vi "Waveform N channels LP pt by pt prefilter.vi"(6 "order":i32=2, 8 "fl":dbl, 10 "fs":dbl, 11 "Array in":waveform(dbl)[](array[waveform])) -> (3 "Array out":waveform(dbl)[](array[waveform]))   [LabVIEW 2013]
uses:
  <vilib>/Analysis/3filter.llb/Filter Passband Type.ctl
  <vilib>/ptbypt/NI_PtbyPt.lvlib
  <vilib>/Analysis/NI_AALBase.lvlib
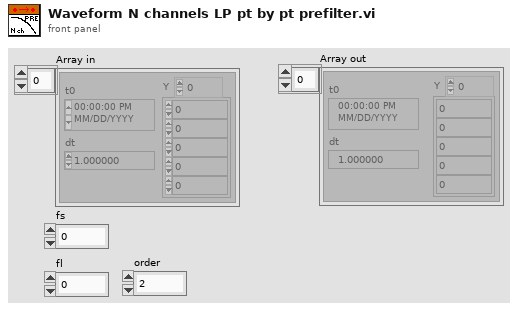
[diagram p1: front panel]
types:
  T1 = typedef "NI_AALBase.lvlib/Filter Passband Type.ctl" = enum32{"Lowpass", "Highpass", "Bandpass", "Bandstop"}
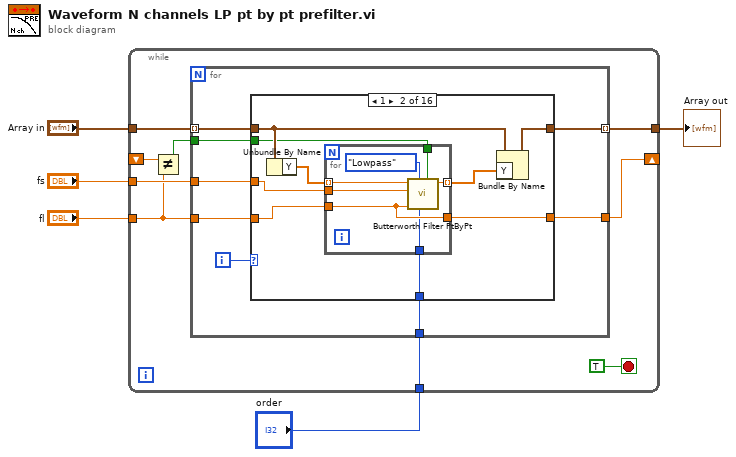
[diagram p0: block diagram]
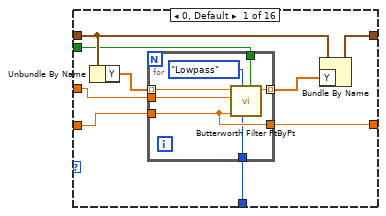
[diagram p2: hidden frame]
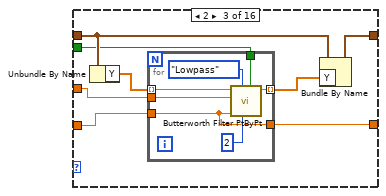
[diagram p3: hidden frame]
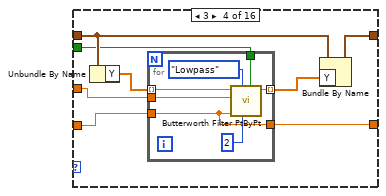
[diagram p4: hidden frame]
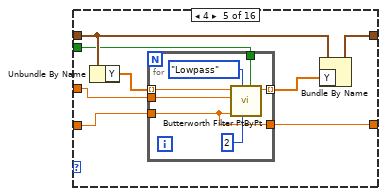
[diagram p5: hidden frame]
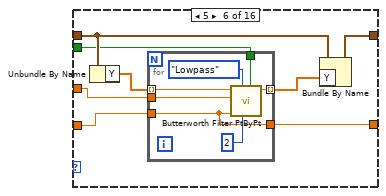
[diagram p6: hidden frame]
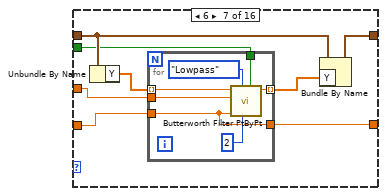
[diagram p7: hidden frame]
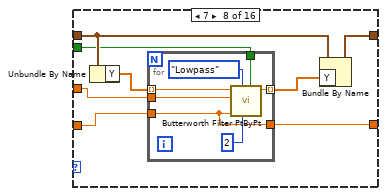
[diagram p8: hidden frame]
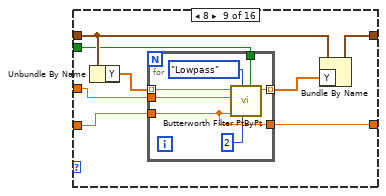
[diagram p9: hidden frame]
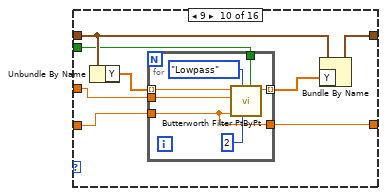
[diagram p10: hidden frame]
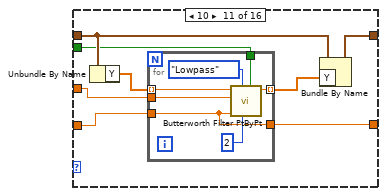
[diagram p11: hidden frame]
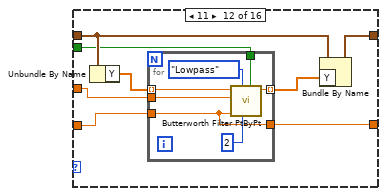
[diagram p12: hidden frame]
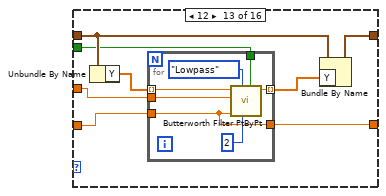
[diagram p13: hidden frame]
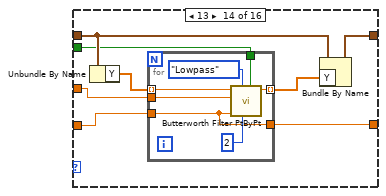
[diagram p14: hidden frame]
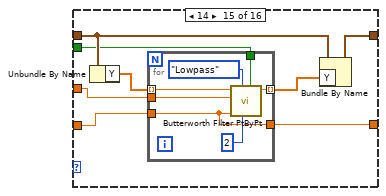
[diagram p15: hidden frame]
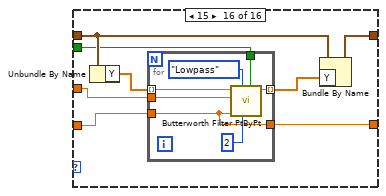
[diagram p16: hidden frame]
diagram:
  n1 = while {
    tunnel: "Array in" -> [w14]
    tunnel: [w13] -> w4
    tunnel: "fs" -> [w10]
    tunnel: "fl" -> [w7]
    shift-right: [w11] -> _
    shift-left: _ -> [w9]
    tunnel: "order" -> [w8]
    stop <- TRUE stop-if-true
    n2 = Not Equal?(x=w9, y=w7) -> (x != y?=w6:bool)
    n3 = for {
      tunnel: w14 -> [w20] mode=indexing
      tunnel: w10 -> [w22]
      tunnel: [w21] -> w13 mode=indexing
      tunnel: w7 -> [w19]
      tunnel: [w17] -> w11
      tunnel: w6 -> [w16]
      tunnel: w8 -> [w15]
      i -> [w18]
      n4 = case shown="1" w18 {
        tunnel: w22 -> [w27 w43 w58 w73 w88 w103 w118 w133 w148 w163 w178 w193 w208 w223 w238 w253]
        tunnel: [w31 w47 w62 w77 w92 w107 w122 w137 w152 w167 w182 w197 w212 w227 w242 w257] -> w21
        tunnel: w20 -> [w29 w45 w60 w75 w90 w105 w120 w135 w150 w165 w180 w195 w210 w225 w240 w255]
        tunnel: [w30 w46 w61 w76 w91 w106 w121 w136 w151 w166 w181 w196 w211 w226 w241 w256] -> w17
        tunnel: w19 -> [w26 w42 w57 w72 w87 w102 w117 w132 w147 w162 w177 w192 w207 w222 w237 w252]
        tunnel: w16 -> [w24 w40 w55 w70 w85 w100 w115 w130 w145 w160 w175 w190 w205 w220 w235 w250]
        tunnel: w15 -> [w23 w39 _ _ _ _ _ _ _ _ _ _ _ _ _ _]
        frame 0, Default {
          n5 = Unbundle By Name(w29) -> ("Y"=w25:dbl[])
          n6 = for {
            tunnel: w25 -> [w38] mode=indexing
            tunnel: w26 -> [w35]
            tunnel: w27 -> [w37]
            tunnel: [w36] -> w28 mode=indexing
            tunnel: [w35] -> w30
            tunnel: w24 -> [w33]
            tunnel: w23 -> [w32]
            n7 = call <vilib>:"Butterworth Filter PtByPt.vi"("initialize"=w33, "order"=w32, "filter type"=Filter_Passband_Type."Lowpass", "low cutoff freq: fl"=w35, "sampling freq: fs"=w37, "x"=w38) -> ("Filtered x"=w36:dbl)  [unwired: 3 in, 1 out]
          }
          n8 = Bundle By Name(cluster=w29, "Y"=w28) -> (w31:waveform(dbl))
        }
        frame 1 {
          n9 = Unbundle By Name(w45) -> ("Y"=w41:dbl[])
          n10 = for {
            tunnel: w41 -> [w54] mode=indexing
            tunnel: w42 -> [w51]
            tunnel: w43 -> [w53]
            tunnel: [w52] -> w44 mode=indexing
            tunnel: [w51] -> w46
            tunnel: w40 -> [w49]
            tunnel: w39 -> [w48]
            n11 = call <vilib>:"Butterworth Filter PtByPt.vi"("initialize"=w49, "order"=w48, "filter type"=Filter_Passband_Type."Lowpass", "low cutoff freq: fl"=w51, "sampling freq: fs"=w53, "x"=w54) -> ("Filtered x"=w52:dbl)  [unwired: 3 in, 1 out]
          }
          n12 = Bundle By Name(cluster=w45, "Y"=w44) -> (w47:waveform(dbl))
        }
        frame 2 {
          n13 = Unbundle By Name(w60) -> ("Y"=w56:dbl[])
          n14 = for {
            tunnel: w56 -> [w69] mode=indexing
            tunnel: w57 -> [w65]
            tunnel: w58 -> [w67]
            tunnel: [w66] -> w59 mode=indexing
            tunnel: [w65] -> w61
            tunnel: w55 -> [w63]
            n15 = call <vilib>:"Butterworth Filter PtByPt.vi"("initialize"=w63, "order"=2, "filter type"=Filter_Passband_Type."Lowpass", "low cutoff freq: fl"=w65, "sampling freq: fs"=w67, "x"=w69) -> ("Filtered x"=w66:dbl)  [unwired: 3 in, 1 out]
          }
          n16 = Bundle By Name(cluster=w60, "Y"=w59) -> (w62:waveform(dbl))
        }
        frame 3 {
          n17 = Unbundle By Name(w75) -> ("Y"=w71:dbl[])
          n18 = for {
            tunnel: w71 -> [w84] mode=indexing
            tunnel: w72 -> [w80]
            tunnel: w73 -> [w82]
            tunnel: [w81] -> w74 mode=indexing
            tunnel: [w80] -> w76
            tunnel: w70 -> [w78]
            n19 = call <vilib>:"Butterworth Filter PtByPt.vi"("initialize"=w78, "order"=2, "filter type"=Filter_Passband_Type."Lowpass", "low cutoff freq: fl"=w80, "sampling freq: fs"=w82, "x"=w84) -> ("Filtered x"=w81:dbl)  [unwired: 3 in, 1 out]
          }
          n20 = Bundle By Name(cluster=w75, "Y"=w74) -> (w77:waveform(dbl))
        }
        frame 4 {
          n21 = Unbundle By Name(w90) -> ("Y"=w86:dbl[])
          n22 = for {
            tunnel: w86 -> [w99] mode=indexing
            tunnel: w87 -> [w95]
            tunnel: w88 -> [w97]
            tunnel: [w96] -> w89 mode=indexing
            tunnel: [w95] -> w91
            tunnel: w85 -> [w93]
            n23 = call <vilib>:"Butterworth Filter PtByPt.vi"("initialize"=w93, "order"=2, "filter type"=Filter_Passband_Type."Lowpass", "low cutoff freq: fl"=w95, "sampling freq: fs"=w97, "x"=w99) -> ("Filtered x"=w96:dbl)  [unwired: 3 in, 1 out]
          }
          n24 = Bundle By Name(cluster=w90, "Y"=w89) -> (w92:waveform(dbl))
        }
        frame 5 {
          n25 = Unbundle By Name(w105) -> ("Y"=w101:dbl[])
          n26 = for {
            tunnel: w101 -> [w114] mode=indexing
            tunnel: w102 -> [w110]
            tunnel: w103 -> [w112]
            tunnel: [w111] -> w104 mode=indexing
            tunnel: [w110] -> w106
            tunnel: w100 -> [w108]
            n27 = call <vilib>:"Butterworth Filter PtByPt.vi"("initialize"=w108, "order"=2, "filter type"=Filter_Passband_Type."Lowpass", "low cutoff freq: fl"=w110, "sampling freq: fs"=w112, "x"=w114) -> ("Filtered x"=w111:dbl)  [unwired: 3 in, 1 out]
          }
          n28 = Bundle By Name(cluster=w105, "Y"=w104) -> (w107:waveform(dbl))
        }
        frame 6 {
          n29 = Unbundle By Name(w120) -> ("Y"=w116:dbl[])
          n30 = for {
            tunnel: w116 -> [w129] mode=indexing
            tunnel: w117 -> [w125]
            tunnel: w118 -> [w127]
            tunnel: [w126] -> w119 mode=indexing
            tunnel: [w125] -> w121
            tunnel: w115 -> [w123]
            n31 = call <vilib>:"Butterworth Filter PtByPt.vi"("initialize"=w123, "order"=2, "filter type"=Filter_Passband_Type."Lowpass", "low cutoff freq: fl"=w125, "sampling freq: fs"=w127, "x"=w129) -> ("Filtered x"=w126:dbl)  [unwired: 3 in, 1 out]
          }
          n32 = Bundle By Name(cluster=w120, "Y"=w119) -> (w122:waveform(dbl))
        }
        frame 7 {
          n33 = Unbundle By Name(w135) -> ("Y"=w131:dbl[])
          n34 = for {
            tunnel: w131 -> [w144] mode=indexing
            tunnel: w132 -> [w140]
            tunnel: w133 -> [w142]
            tunnel: [w141] -> w134 mode=indexing
            tunnel: [w140] -> w136
            tunnel: w130 -> [w138]
            n35 = call <vilib>:"Butterworth Filter PtByPt.vi"("initialize"=w138, "order"=2, "filter type"=Filter_Passband_Type."Lowpass", "low cutoff freq: fl"=w140, "sampling freq: fs"=w142, "x"=w144) -> ("Filtered x"=w141:dbl)  [unwired: 3 in, 1 out]
          }
          n36 = Bundle By Name(cluster=w135, "Y"=w134) -> (w137:waveform(dbl))
        }
        frame 8 {
          n37 = Unbundle By Name(w150) -> ("Y"=w146:dbl[])
          n38 = for {
            tunnel: w146 -> [w159] mode=indexing
            tunnel: w147 -> [w155]
            tunnel: w148 -> [w157]
            tunnel: [w156] -> w149 mode=indexing
            tunnel: [w155] -> w151
            tunnel: w145 -> [w153]
            n39 = call <vilib>:"Butterworth Filter PtByPt.vi"("initialize"=w153, "order"=2, "filter type"=Filter_Passband_Type."Lowpass", "low cutoff freq: fl"=w155, "sampling freq: fs"=w157, "x"=w159) -> ("Filtered x"=w156:dbl)  [unwired: 3 in, 1 out]
          }
          n40 = Bundle By Name(cluster=w150, "Y"=w149) -> (w152:waveform(dbl))
        }
        frame 9 {
          n41 = Unbundle By Name(w165) -> ("Y"=w161:dbl[])
          n42 = for {
            tunnel: w161 -> [w174] mode=indexing
            tunnel: w162 -> [w170]
            tunnel: w163 -> [w172]
            tunnel: [w171] -> w164 mode=indexing
            tunnel: [w170] -> w166
            tunnel: w160 -> [w168]
            n43 = call <vilib>:"Butterworth Filter PtByPt.vi"("initialize"=w168, "order"=2, "filter type"=Filter_Passband_Type."Lowpass", "low cutoff freq: fl"=w170, "sampling freq: fs"=w172, "x"=w174) -> ("Filtered x"=w171:dbl)  [unwired: 3 in, 1 out]
          }
          n44 = Bundle By Name(cluster=w165, "Y"=w164) -> (w167:waveform(dbl))
        }
        frame 10 {
          n45 = Unbundle By Name(w180) -> ("Y"=w176:dbl[])
          n46 = for {
            tunnel: w176 -> [w189] mode=indexing
            tunnel: w177 -> [w185]
            tunnel: w178 -> [w187]
            tunnel: [w186] -> w179 mode=indexing
            tunnel: [w185] -> w181
            tunnel: w175 -> [w183]
            n47 = call <vilib>:"Butterworth Filter PtByPt.vi"("initialize"=w183, "order"=2, "filter type"=Filter_Passband_Type."Lowpass", "low cutoff freq: fl"=w185, "sampling freq: fs"=w187, "x"=w189) -> ("Filtered x"=w186:dbl)  [unwired: 3 in, 1 out]
          }
          n48 = Bundle By Name(cluster=w180, "Y"=w179) -> (w182:waveform(dbl))
        }
        frame 11 {
          n49 = Unbundle By Name(w195) -> ("Y"=w191:dbl[])
          n50 = for {
            tunnel: w191 -> [w204] mode=indexing
            tunnel: w192 -> [w200]
            tunnel: w193 -> [w202]
            tunnel: [w201] -> w194 mode=indexing
            tunnel: [w200] -> w196
            tunnel: w190 -> [w198]
            n51 = call <vilib>:"Butterworth Filter PtByPt.vi"("initialize"=w198, "order"=2, "filter type"=Filter_Passband_Type."Lowpass", "low cutoff freq: fl"=w200, "sampling freq: fs"=w202, "x"=w204) -> ("Filtered x"=w201:dbl)  [unwired: 3 in, 1 out]
          }
          n52 = Bundle By Name(cluster=w195, "Y"=w194) -> (w197:waveform(dbl))
        }
        frame 12 {
          n53 = Unbundle By Name(w210) -> ("Y"=w206:dbl[])
          n54 = for {
            tunnel: w206 -> [w219] mode=indexing
            tunnel: w207 -> [w215]
            tunnel: w208 -> [w217]
            tunnel: [w216] -> w209 mode=indexing
            tunnel: [w215] -> w211
            tunnel: w205 -> [w213]
            n55 = call <vilib>:"Butterworth Filter PtByPt.vi"("initialize"=w213, "order"=2, "filter type"=Filter_Passband_Type."Lowpass", "low cutoff freq: fl"=w215, "sampling freq: fs"=w217, "x"=w219) -> ("Filtered x"=w216:dbl)  [unwired: 3 in, 1 out]
          }
          n56 = Bundle By Name(cluster=w210, "Y"=w209) -> (w212:waveform(dbl))
        }
        frame 13 {
          n57 = Unbundle By Name(w225) -> ("Y"=w221:dbl[])
          n58 = for {
            tunnel: w221 -> [w234] mode=indexing
            tunnel: w222 -> [w230]
            tunnel: w223 -> [w232]
            tunnel: [w231] -> w224 mode=indexing
            tunnel: [w230] -> w226
            tunnel: w220 -> [w228]
            n59 = call <vilib>:"Butterworth Filter PtByPt.vi"("initialize"=w228, "order"=2, "filter type"=Filter_Passband_Type."Lowpass", "low cutoff freq: fl"=w230, "sampling freq: fs"=w232, "x"=w234) -> ("Filtered x"=w231:dbl)  [unwired: 3 in, 1 out]
          }
          n60 = Bundle By Name(cluster=w225, "Y"=w224) -> (w227:waveform(dbl))
        }
        frame 14 {
          n61 = Unbundle By Name(w240) -> ("Y"=w236:dbl[])
          n62 = for {
            tunnel: w236 -> [w249] mode=indexing
            tunnel: w237 -> [w245]
            tunnel: w238 -> [w247]
            tunnel: [w246] -> w239 mode=indexing
            tunnel: [w245] -> w241
            tunnel: w235 -> [w243]
            n63 = call <vilib>:"Butterworth Filter PtByPt.vi"("initialize"=w243, "order"=2, "filter type"=Filter_Passband_Type."Lowpass", "low cutoff freq: fl"=w245, "sampling freq: fs"=w247, "x"=w249) -> ("Filtered x"=w246:dbl)  [unwired: 3 in, 1 out]
          }
          n64 = Bundle By Name(cluster=w240, "Y"=w239) -> (w242:waveform(dbl))
        }
        frame 15 {
          n65 = Unbundle By Name(w255) -> ("Y"=w251:dbl[])
          n66 = for {
            tunnel: w251 -> [w264] mode=indexing
            tunnel: w252 -> [w260]
            tunnel: w253 -> [w262]
            tunnel: [w261] -> w254 mode=indexing
            tunnel: [w260] -> w256
            tunnel: w250 -> [w258]
            n67 = call <vilib>:"Butterworth Filter PtByPt.vi"("initialize"=w258, "order"=2, "filter type"=Filter_Passband_Type."Lowpass", "low cutoff freq: fl"=w260, "sampling freq: fs"=w262, "x"=w264) -> ("Filtered x"=w261:dbl)  [unwired: 3 in, 1 out]
          }
          n68 = Bundle By Name(cluster=w255, "Y"=w254) -> (w257:waveform(dbl))
        }
      }
    }
  }
  "Array out" <- w4
